vi "Green Board DC Bus Test_v2.vi"(8 "error in (no error)":errorcluster, 10 "HMP VISA":refnum<visa-resource-name>, 11 "Control Board VISA":refnum<visa-resource-name>) -> (0 "error out":errorcluster, 2 "Voltage DC charged":dbl, 3 "Voltage (0V)":dbl)   [LabVIEW 2022 SP3]
uses:
  Serial Board Com/ADCSelector GB.ctl
  HMP4000 Communication/HMP4040_ChannelControlAutomatic.ctl
panel:
  out "Message OUT":string
  in  "Message IN":string
  out "Pass/Fail":bool
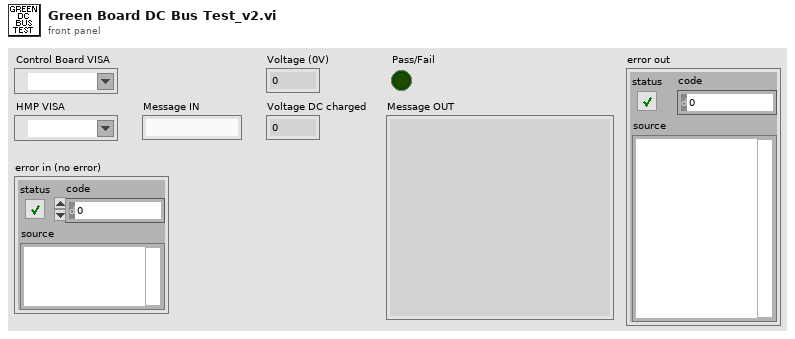
[diagram p1: front panel]
types:
  T1 = typedef "HMP4040_ChannelControlAutomatic.ctl" = enum16{"Off", "Control Power", "HMP2020 Control + DC32V", "HMP2020 Control + DC8V", "HMP4040 Control + DC32V", "HMP4040 Control +DC8V", "HMP4040 Ch2 24V 4A"}
  T2 = typedef "ADCSelector GB.ctl" = enum16{"INVA_ISENSE_U", "INVA_ISENSE_V", "INVA_ISENSE_W", "INVA_UDC", "INVA_TEMP", "HB_ISENSE", "AUX_ISENSE_U", "AUX_ISENSE_V", "AUX_ISENSE_W", "VLINE_AB", "VLINE_BC", "VLINE_CA", "REF_1P5V", "VSENSE_POS_24V", "VSENSE_POS_5V", "VSENSE_NEG_15V", "TEST_POINT", "INVB_ISENSE_U", "INVB_ISENSE_V", "INVB_ISENSE_W", "INVB_UDC", "INVB_TEMP", "HB_TEMP", "AUXA_TEMP", "AUXB_TEMP", "AUXC_TEMP", "VOUT_AB", "VOUT_BC", "VOUT_CA", "REF_2P5V", "VSENSE_POS_15V", "VSENSE_POS_3P3V", "NET_ANALYZER"}
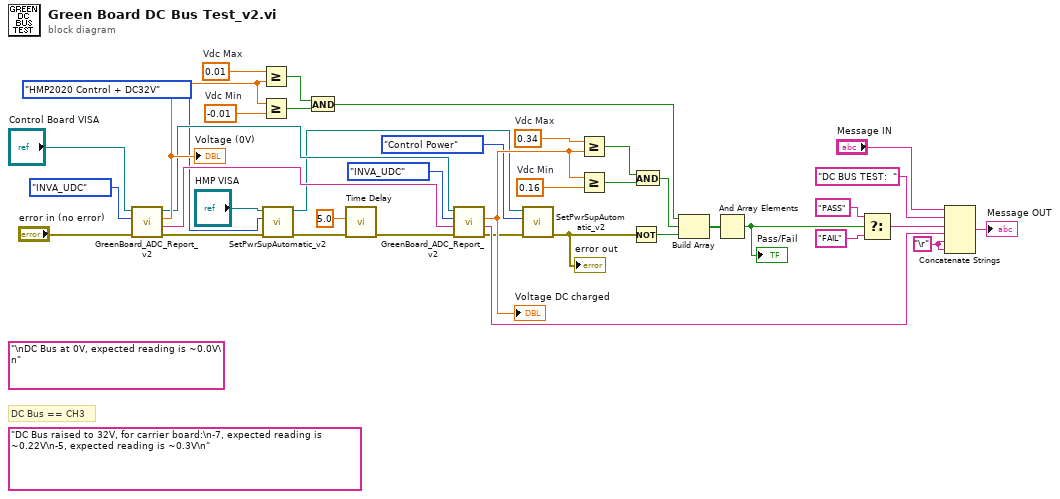
[diagram p0: block diagram]
diagram:
  (unwired) "DC Bus raised to 32V, for carrier board:\n-7, expected reading is ~0.22V\n-5, expected reading is ~0.3V\n"
  w18 = "\r"
  (unwired) "\nDC Bus at 0V, expected reading is ~0.0V\n"
  w31 = -0.01  # Vdc Min
  w30 = 0.01  # Vdc Max
  w38 = 0.16  # Vdc Min
  w39 = 0.34  # Vdc Max
  # "DC Bus == CH3"
  n1 = call "GreenBoard_ADC_Report_v2.vi"("error in (no error)"="error in (no error)", "Green Board Enum"=ADCSelector_GB."INVA_UDC", "ControlBoard VISA"="Control Board VISA") -> ("error out"=w29:errorcluster, "Message OUT"=w7:string, "Result"=w12:dbl, "VISA Refnum out"=w8:refnum<visa-resource-name>)  [unwired: 5 in]
  "Voltage (0V)" <- w12
  n2 = Greater Or Equal?(x=w30, y=w12) -> (x >= y?=w32:bool)
  n3 = Greater Or Equal?(x=w12, y=w31) -> (x >= y?=w33:bool)
  n4 = call "SetPwrSupAutomatic_v2.vi"("error in (no error)"=w29, "Enum"=HMP4040_ChannelControlAutomatic."HMP2020 Control + DC32V", "HMP VISA"="HMP VISA") -> ("error out"=w35:errorcluster, "HMP VISA Out"=w4:refnum<visa-resource-name>)  [unwired: 7 in]
  n5 = And(x=w32, y=w33) -> (x .and. y?=w16:bool)
  n6 = call "Time Delay"("error in (no error)"=w35, "Delay Time (s)"=5.0) -> ("error out"=w34:errorcluster)  [unwired: 9 in]
  n7 = call "GreenBoard_ADC_Report_v2.vi"("error in (no error)"=w34, "Message IN"=w7, "Green Board Enum"=ADCSelector_GB."INVA_UDC", "ControlBoard VISA"=w8) -> ("error out"=w3:errorcluster, "Message OUT"=w26:string, "Result"=w11:dbl)  [unwired: 4 in, 1 out]
  "Voltage DC charged" <- w11
  n8 = call "SetPwrSupAutomatic_v2.vi"("error in (no error)"=w3, "Enum"=HMP4040_ChannelControlAutomatic."Control Power", "HMP VISA"=w4) -> ("error out"=w2:errorcluster)  [unwired: 7 in, 1 out]
  "error out" <- w2
  n9 = Greater Or Equal?(x=w39, y=w11) -> (x >= y?=w37:bool)
  n10 = Greater Or Equal?(x=w11, y=w38) -> (x >= y?=w36:bool)
  n11 = Not(x=w2) -> (.not. x?=w28:bool)
  n12 = And(x=w37, y=w36) -> (x .and. y?=w17:bool)
  n13 = Build Array(w16, w17, w28) -> (w27:bool[])
  n14 = And Array Elements(Boolean array=w27) -> (logical AND=w20:bool)
  "Pass/Fail" <- w20
  n15 = Select(t="PASS", s=w20, f="FAIL") -> (s? t:f=w19:string)
  n16 = Concatenate Strings("Message IN", "DC BUS TEST:  " ("string"), w19, w26, w18, w18) -> (→"Message OUT":string)
